vi "Check Items Existence In memory.vi"(8 "error in (no error)":errorcluster, 11 "Methods to be Wrapped":string[](array[string])) -> (0 "error out":errorcluster, 3 "Notify?":bool)   [LabVIEW 2020, in "WebServiceImporter.lvlib" / "Main Panel.lvlib" / "Select Methods.lvlib"]
uses:
  <vilib>/Platform/WebService/Main Panel/Pages/Select Methods/Select Methods.lvlib
  <vilib>/Platform/WebService/Global/Const Strings.vi
  <vilib>/Platform/WebService/VI Generator/VI Generator.lvlib
  <vilib>/Platform/WebService/WebServiceImporter.lvlib
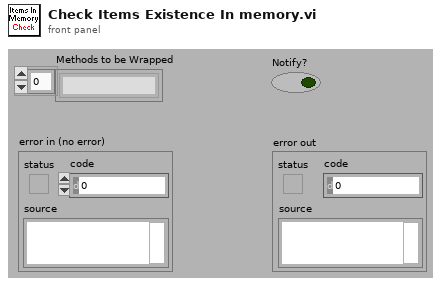
[diagram p1: front panel]
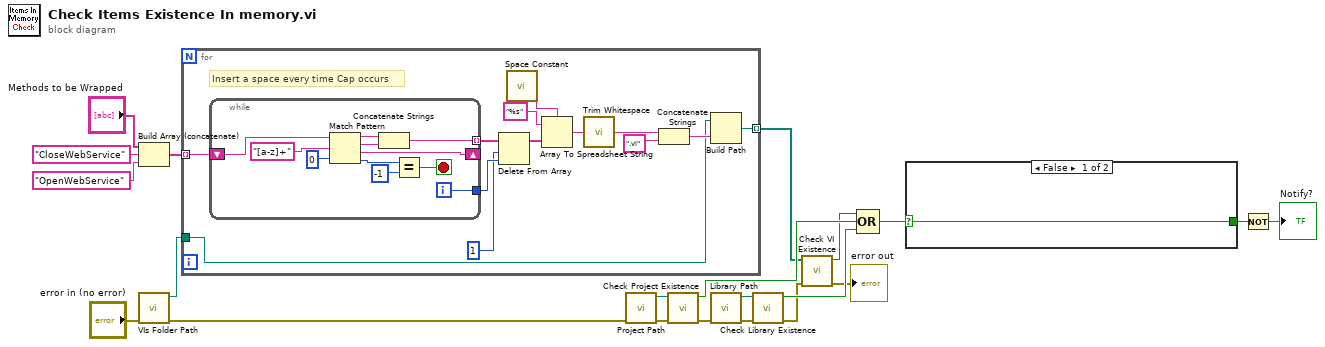
[diagram p0: block diagram]
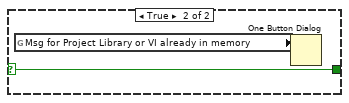
[diagram p2: hidden frame]
diagram:
  n1 = Build Array (concatenate)("Methods to be Wrapped", "CloseWebService", "OpenWebService" ("element")) -> (w9:string[])
  n2 = call <vilib>:"VIs Folder Path.vi"("error in (no error)"="error in (no error)") -> ("error out"=w10:errorcluster, "Path 2"=w5:path)  [unwired: 2 in, 7 out]
  n3 = for {
    tunnel: w9 -> [w23] mode=indexing
    tunnel: [w32] -> w11 mode=indexing
    tunnel: w5 -> [w31]
    # "Insert a space every time Cap occurs"
    n4 = while {
      shift-right: [w41] -> _
      shift-left: w23 -> [w43]
      tunnel: [w37] -> w25 mode=indexing
      tunnel: [w35] -> w26
      i -> [w35]
      stop <- w44 stop-if-true
      n5 = Match Pattern(string=w43, regular expression="[a-z]+", offset (0)=0) -> (before substring=w39:string, match substring=w38:string, after substring=w41:string, offset past match=w36:i32)
      n6 = Concatenate Strings(w39, w38) -> (w37:string)
      n7 = Equal?(x=w36, y=-1) -> (x = y?=w44:bool)
    }
    n8 = Delete From Array(array=w25, length=1, index=w26) -> (array with subset deleted=w29:string[])  [unwired: 1 out]
    n9 = call <vilib>:"Space Constant.vi"() -> ("String"=w28:string)
    n10 = Array To Spreadsheet String(delimiter (Tab)=w28, array=w29, 3:"%s" ("格式字符串")) -> (spreadsheet string=w30:string)
    n11 = call <vilib>:"Trim Whitespace.vi"("string"=w30) -> ("trimmed string"=w22:string)  [unwired: 1 in]
    n12 = Concatenate Strings(w22, ".vi" ("string")) -> (w34:string)
    n13 = Build Path(base path=w31, name or relative path=w34) -> (appended path=w32:path)
  }
  n14 = call <vilib>:"Project Path.vi"("error in (no error)"=w10) -> ("error out"=w12:errorcluster, "Path (out)"=w4:path)  [unwired: 2 in, 7 out]
  n15 = call <vilib>:"Check Project Existence.vi"("error in (no error)"=w12, "Proj Path"=w4) -> ("error out"=w13:errorcluster, "Find Existence?"=w20:bool)  [unwired: 1 in, 7 out]
  n16 = call <vilib>:"Library Path.vi"("error in (no error)"=w13) -> ("error out"=w15:errorcluster, "Path (out)"=w14:path)  [unwired: 2 in, 7 out]
  n17 = call <vilib>:"Check Library Existence.vi"("error in (no error)"=w15, "Lib Path"=w14) -> ("error out"=w18:errorcluster, "Existence?"=w21:bool)  [unwired: 8 out]
  n18 = call <vilib>:"Check VI Existence.vi"("error in (no error)"=w18, "VIs Path"=w11) -> ("error out"=→"error out":errorcluster, "Existence?"=w1:bool)  [unwired: 8 out]
  n19 = Compound Arithmetic op=OR(w1, w20, w21) -> (w16:bool)
  n20 = case shown="False" w16 {
    selector: w16 -> [w46 w48]
    tunnel: [w46 w48] -> w17
    frame False {
    }
    frame True {
      n21 = global read "Const Strings.vi" "Msg for Project Library or VI already in memory"() -> (w47:string)
      n22 = One Button Dialog(message=w47) -> ()  [unwired: 2 out]
    }
  }
  n23 = Not(x=w17) -> (.not. x?=→"Notify?":bool)
